vi "Chroma 617xx Driver GPIB-VISA-RW.vi"(0 "VISA resource name":refnum<visa-resource-name>="CHROMA", 1 "L1 Adjusted":string, 2 "L2 Adjusted":string, 5 "Chroma Power Select":T1, 7 "Use Adjusted Voltage":bool, 9 "Write Buffer":string="SENS:DATA?", 11 "error in (no error)":errorcluster) -> (6 "Read Array":string[](array[string]), 15 "error out":errorcluster)   [LabVIEW 2016]
doc: "This example requires NI-488.2 and NI-VISA to be installed on the system. The example shows how to communicate with a GPIB instrument using VISA reads, writes, and formatting functions on the returned data. This example will work using an NI Instrument Simulator or other instrument that has similar behavior."
uses:
  Type Definition/Chroma Driver Select.ctl
  <vilib>/Instr/_visa.llb/VISA Open Access Mode.ctl
panel:
  out "Array":errorcluster[](array[cluster])
  out "Success":bool
  out "Read Buffer":string
  # "Voltage \nPower\nCurrent \nState\nPhase\nError?"
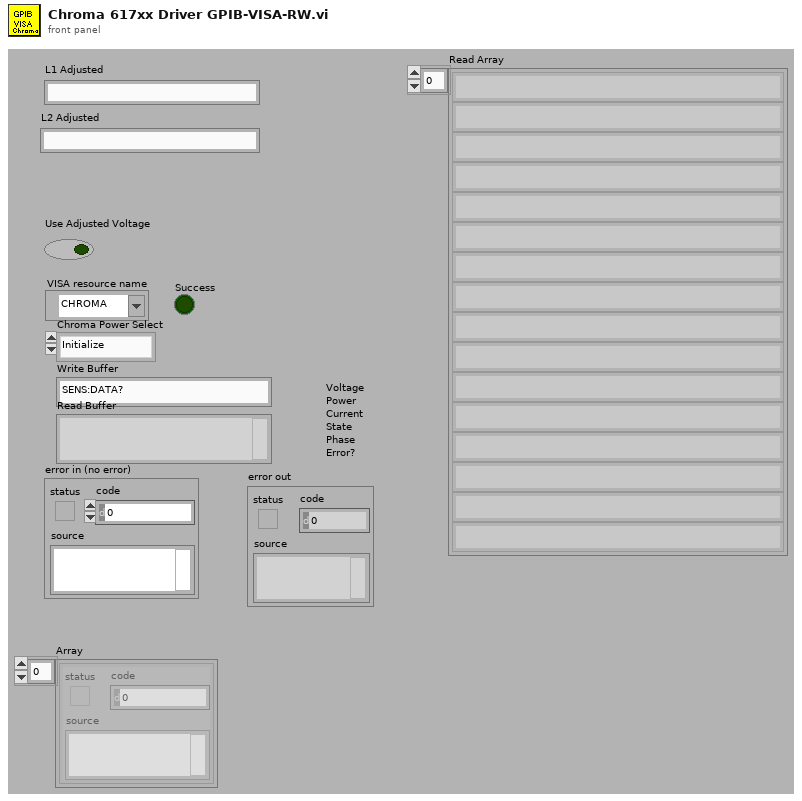
[diagram p1: front panel]
types:
  T1 = typedef "Chroma Driver Select.ctl" = enum16{"Initialize", "Output On 120", "Output On 240", "Output On 208", "Output Off", "Status", "Send Command", "Track Current"}
  T2 = typedef "VISA Open Access Mode.ctl" = u32
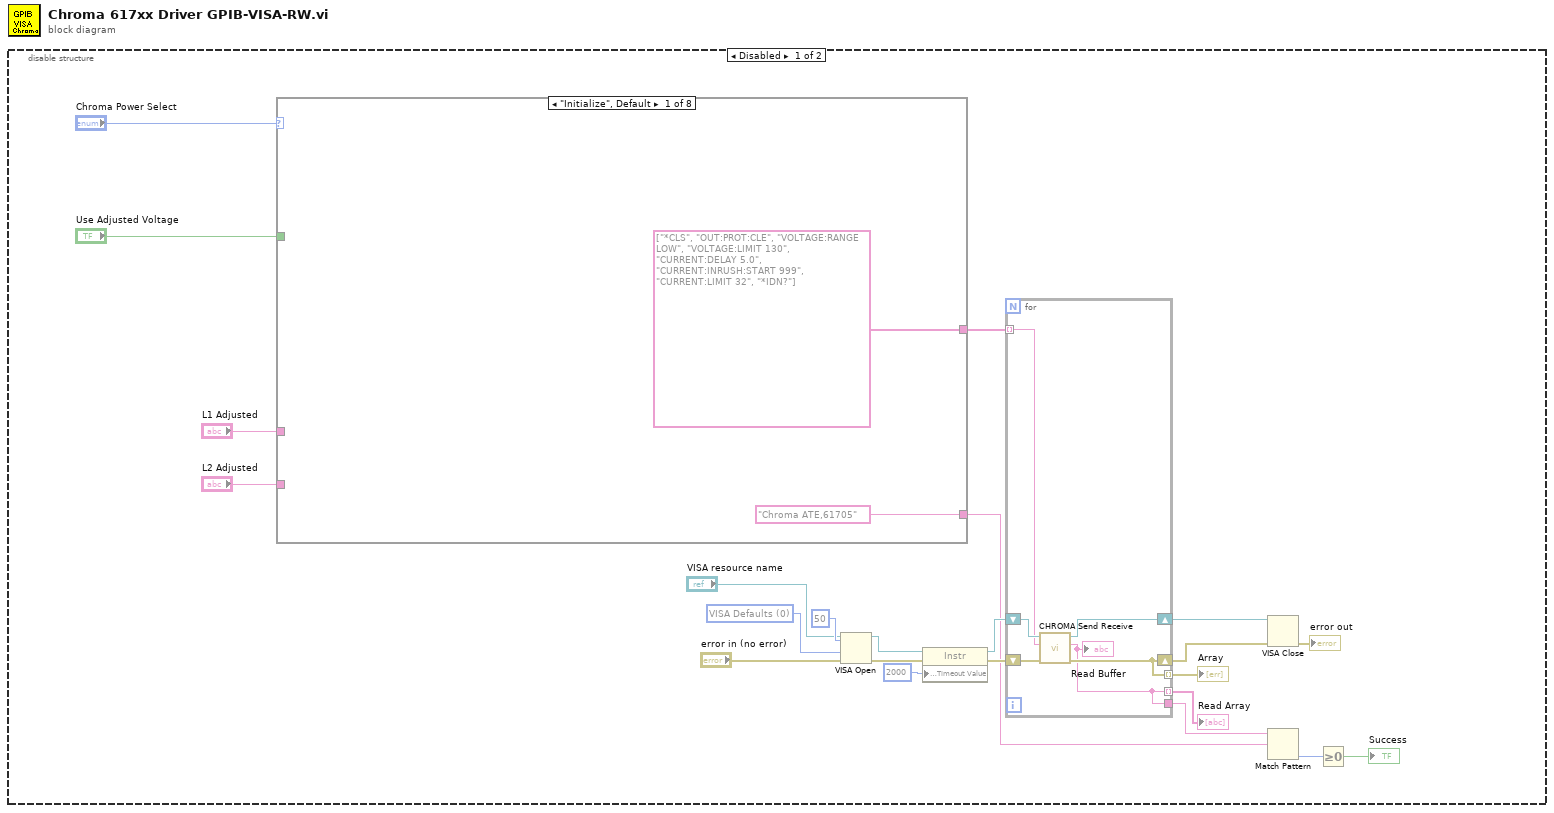
[diagram p0: block diagram]
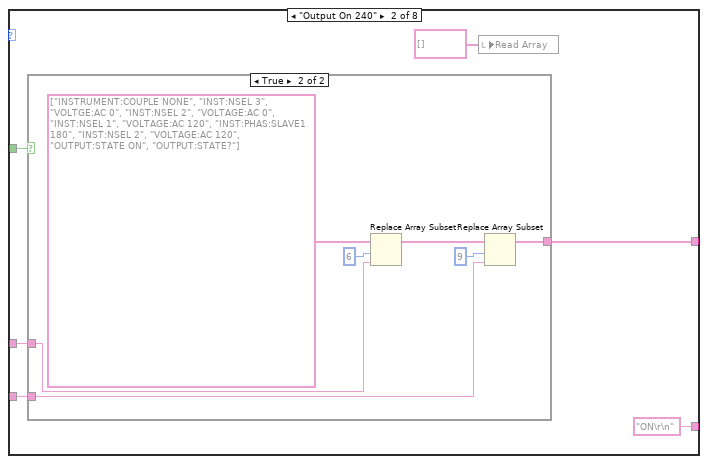
[diagram p2: hidden frame]
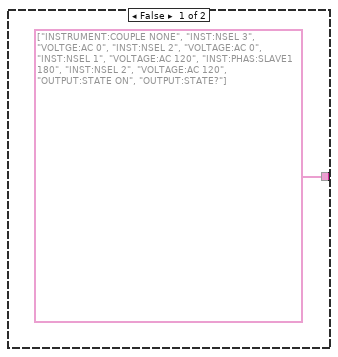
[diagram p3: hidden frame]
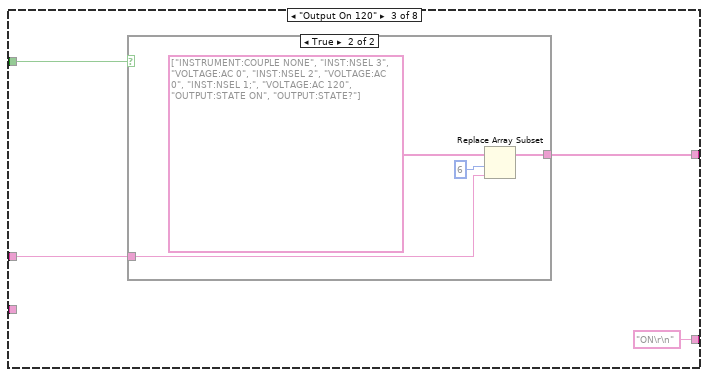
[diagram p4: hidden frame]
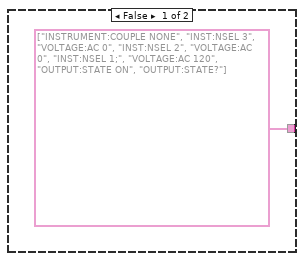
[diagram p5: hidden frame]
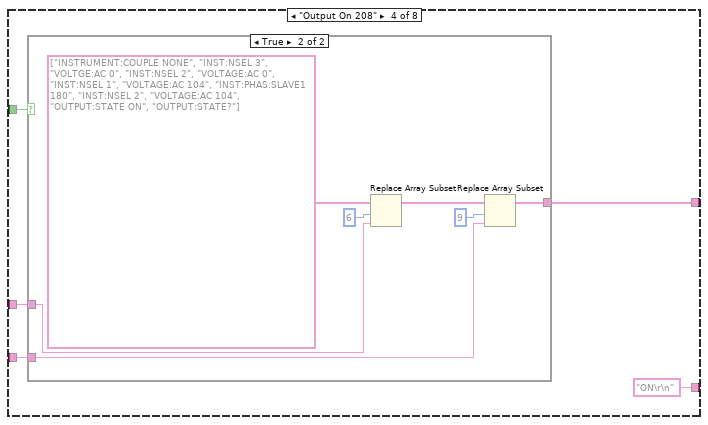
[diagram p6: hidden frame]
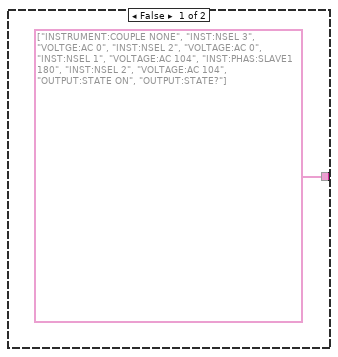
[diagram p7: hidden frame]
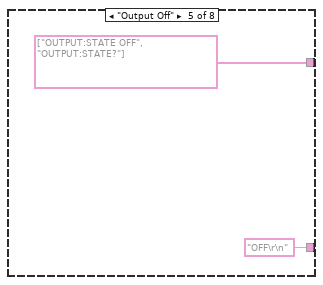
[diagram p8: hidden frame]
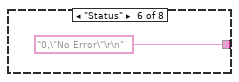
[diagram p9: hidden frame]
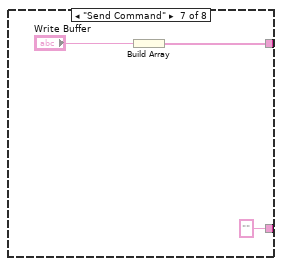
[diagram p10: hidden frame]
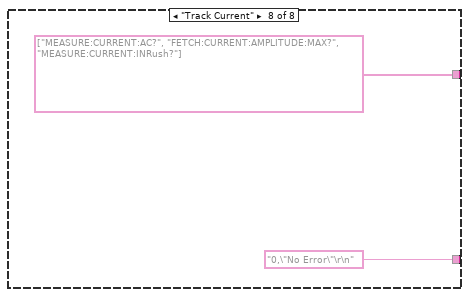
[diagram p11: hidden frame]
diagram:
  n1 = disable-structure shown="Disabled" {
    frame Disabled {
      w17 = T2 0 items=["VISA Defaults"=0, "Exclusive Lock"=1, "Load Configured Settings"=4] ("Access Mode")
      n2 = case shown="\"Initialize\", Default" "Chroma Power Select" {
        tunnel: [string[] ["*CLS", "OUT:PROT:CLE", "VOLTAGE:RANGE LOW", "VOLTAGE:LIMIT 130", "CURRENT:DELAY 5.0", "CURRENT:INRUSH:START 999", "CURRENT:LIMIT 32", "*IDN?"] w35 w48 w58 string[] ["OUTPUT:STATE OFF", "OUTPUT:STATE?"] _ w73 string[] ["MEASURE:CURRENT:AC?", "FETCH:CURRENT:AMPLITUDE:MAX?", "MEASURE:CURRENT:INRush?"]] -> w13
        tunnel: ["Chroma ATE,61705" ("string to write") "ON\r\n" ("read buffer") "ON\r\n" ("read buffer") "ON\r\n" ("read buffer") "OFF\r\n" ("read buffer") "0,\"No Error\"\r\n" ("string to write") "" ("Response") "0,\"No Error\"\r\n" ("string to write")] -> w4
        tunnel: "Use Adjusted Voltage" -> [_ w34 w47 w55 _ _ _ _]
        tunnel: "L1 Adjusted" -> [_ w33 w46 w56 _ _ _ _]
        tunnel: "L2 Adjusted" -> [_ w32 _ w57 _ _ _ _]
        frame "Initialize", Default {
        }
        frame "Output On 240" {
          n3 = case shown="True" w34 {
            tunnel: [string[] ["INSTRUMENT:COUPLE NONE", "INST:NSEL 3", "VOLTGE:AC 0", "INST:NSEL 2", "VOLTAGE:AC 0", "INST:NSEL 1", "VOLTAGE:AC 120", "INST:PHAS:SLAVE1 180", "INST:NSEL 2", "VOLTAGE:AC 120", "OUTPUT:STATE ON", "OUTPUT:STATE?"] w43] -> w35
            tunnel: w33 -> [_ w42]
            tunnel: w32 -> [_ w41]
            frame False {
            }
            frame True {
              n4 = Replace Array Subset(array=string[] ["INSTRUMENT:COUPLE NONE", "INST:NSEL 3", "VOLTGE:AC 0", "INST:NSEL 2", "VOLTAGE:AC 0", "INST:NSEL 1", "VOLTAGE:AC 120", "INST:PHAS:SLAVE1 180", "INST:NSEL 2", "VOLTAGE:AC 120", "OUTPUT:STATE ON", "OUTPUT:STATE?"], new element=w42, index=6) -> (w44:string[])
              n5 = Replace Array Subset(array=w44, new element=w41, index=9) -> (w43:string[])
            }
          }
          n6 = local write "Read Array"(string[] [] ("Read Array")) -> ()
        }
        frame "Output On 120" {
          n7 = case shown="True" w47 {
            tunnel: [string[] ["INSTRUMENT:COUPLE NONE", "INST:NSEL 3", "VOLTAGE:AC 0", "INST:NSEL 2", "VOLTAGE:AC 0", "INST:NSEL 1;", "VOLTAGE:AC 120", "OUTPUT:STATE ON", "OUTPUT:STATE?"] w52] -> w48
            tunnel: w46 -> [_ w53]
            frame False {
            }
            frame True {
              n8 = Replace Array Subset(array=string[] ["INSTRUMENT:COUPLE NONE", "INST:NSEL 3", "VOLTAGE:AC 0", "INST:NSEL 2", "VOLTAGE:AC 0", "INST:NSEL 1;", "VOLTAGE:AC 120", "OUTPUT:STATE ON", "OUTPUT:STATE?"], new element=w53, index=6) -> (w52:string[])
            }
          }
        }
        frame "Output On 208" {
          n9 = case shown="True" w55 {
            tunnel: [string[] ["INSTRUMENT:COUPLE NONE", "INST:NSEL 3", "VOLTGE:AC 0", "INST:NSEL 2", "VOLTAGE:AC 0", "INST:NSEL 1", "VOLTAGE:AC 104", "INST:PHAS:SLAVE1 180", "INST:NSEL 2", "VOLTAGE:AC 104", "OUTPUT:STATE ON", "OUTPUT:STATE?"] w61] -> w58
            tunnel: w57 -> [_ w66]
            tunnel: w56 -> [_ w65]
            frame False {
            }
            frame True {
              n10 = Replace Array Subset(array=string[] ["INSTRUMENT:COUPLE NONE", "INST:NSEL 3", "VOLTGE:AC 0", "INST:NSEL 2", "VOLTAGE:AC 0", "INST:NSEL 1", "VOLTAGE:AC 104", "INST:PHAS:SLAVE1 180", "INST:NSEL 2", "VOLTAGE:AC 104", "OUTPUT:STATE ON", "OUTPUT:STATE?"], new element=w65, index=6) -> (w62:string[])
              n11 = Replace Array Subset(array=w62, new element=w66, index=9) -> (w61:string[])
            }
          }
        }
        frame "Output Off" {
        }
        frame "Status" {
        }
        frame "Send Command" {
          n12 = Build Array("Write Buffer") -> (w73:string[])
        }
        frame "Track Current" {
        }
      }
      n13 = VISA Open(timeout (0)=u32 50 ("VISA Open timeout (0)"), access mode=w17, error in (no error)="error in (no error)", VISA resource name="VISA resource name") -> (VISA resource name=w19:refnum<visa-resource-name>, error out=w18:errorcluster)  [unwired: 1 in]
      n14 = property class="Instr"(reference=w19, error in=w18, "General Settings:Timeout Value"=u32 2000) -> (reference out=w15:refnum<visa-resource-name>, error out=w16:errorcluster)
      n15 = for {
        tunnel: w13 -> [w26] mode=indexing
        shift-right: [w29] -> w23
        shift-left: w15 -> [w27]
        shift-right: [w25] -> w22
        shift-left: w16 -> [w28]
        tunnel: [w24] -> w10 mode=indexing
        tunnel: [w24] -> w5
        tunnel: [w25] -> w9 mode=indexing
        n16 = call "CHROMA Send Receive.vi"("error in (no error)"=w28, "Send Command"=w26, "CHROMA VISA In"=w27) -> ("error out"=w25:errorcluster, "read buffer"=w24:string, "CHROMA VISA Out"=w29:refnum<visa-resource-name>)  [unwired: 6 in]
        "Read Buffer" <- w24
      }
      "Read Array" <- w10
      "Array" <- w9
      n17 = VISA Close(VISA resource name=w23, error in (no error)=w22) -> (error out=→"error out":errorcluster)
      n18 = Match Pattern(string=w5, regular expression=w4) -> (offset past match=w7:i32)  [unwired: 1 in, 3 out]
      n19 = Greater Or Equal To 0?(x=w7) -> (x >= 0?=→"Success":bool)
    }
    frame Enabled {
    }
  }
